vi "tm_inputtriggersource_40.vi"(8 "error in (no error)":errorcluster, 9 "External Options":cluster{"Polarity":i32, "Delay":dbl}={"Polarity"=1, "Delay"=0.0} {"Polarity" items=["Negative"=1, "Positive"=2]}, 10 "Source":i32(ring)=1 items=["Internal"=1, "External"=2, "Software"=3, "Master Pulse"=4], 11 "Handle in":u32) -> (0 "error out":errorcluster, 3 "Handle out":u32)   [LabVIEW 2023]
uses:
  tmcamcon.dll
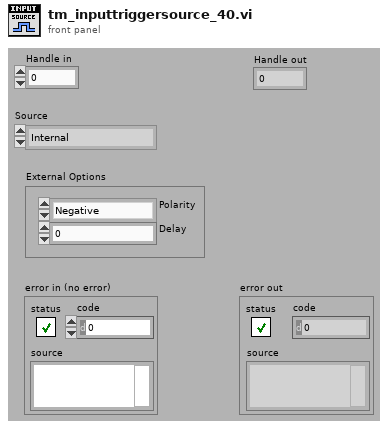
[diagram p1: front panel]
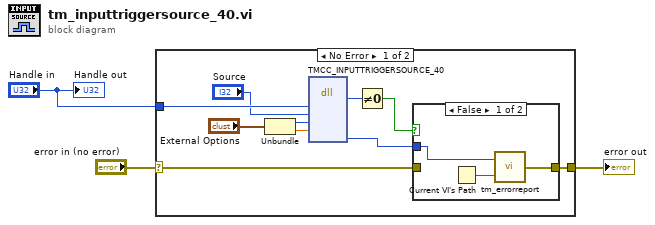
[diagram p0: block diagram]
diagram:
  n1 = case shown="No Error" "error in (no error)" {
    selector: "error in (no error)" -> [w11 w18]
    tunnel: [w8 w18] -> w2
    tunnel: "Handle in" -> [w12 _]
    frame No Error {
      n2 = Unbundle("External Options") -> ("Polarity"=w5:i32, "Delay"=w4:dbl)
      n3 = dll-call lib="tmcamcon.dll" fn="TMCC_INPUTTRIGGERSOURCE_40"("HDCAM"=w12, "source"="Source", "polarity"=w5, "delay"=w4) -> ("return type"=w13:u32, "Erval"=w10:i32)  [unwired: 8 in, 2 out]
      n4 = Not Equal To 0?(x=w13) -> (x != 0?=w9:bool)
      n5 = case shown="False" w9 {
        tunnel: w11 -> [_ w17]
        tunnel: [w15 w17] -> w8
        tunnel: w10 -> [w14 _]
        frame False {
          n6 = Current VI's Path() -> (path=w16:path)
          n7 = call "tm_errorreport.vi"("Source"=w16, "Error"=w14) -> ("error out"=w15:errorcluster)
        }
        frame True {
        }
      }
    }
    frame Error {
    }
  }
  "error out" <- w2
  "Handle out" <- "Handle in"
